vi "ISO8601 TimeString to Timestamp.vi"(9 "Strict ISO? (T)":bool=TRUE, 10 "Date (today)":timestamp, 11 "ISO8601 Time String":string) -> (1 "valid?":bool, 3 "Timestamp":timestamp)   [LabVIEW 2024]
uses:
  <vilib>/regexp/Match Regular Expression.xnode
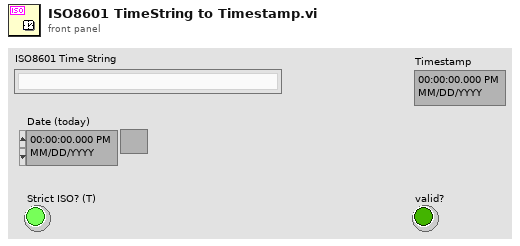
[diagram p1: front panel]
types:
  T1 = typedef "LVDateTimeRec.ctl" = cluster{"fractional second":dbl, "second":i32, "minute":i32, "hour":i32, "day of month":i32, "month":i32, "year":i32, "day of week":i32, "day of year":i32, "DST":i32}
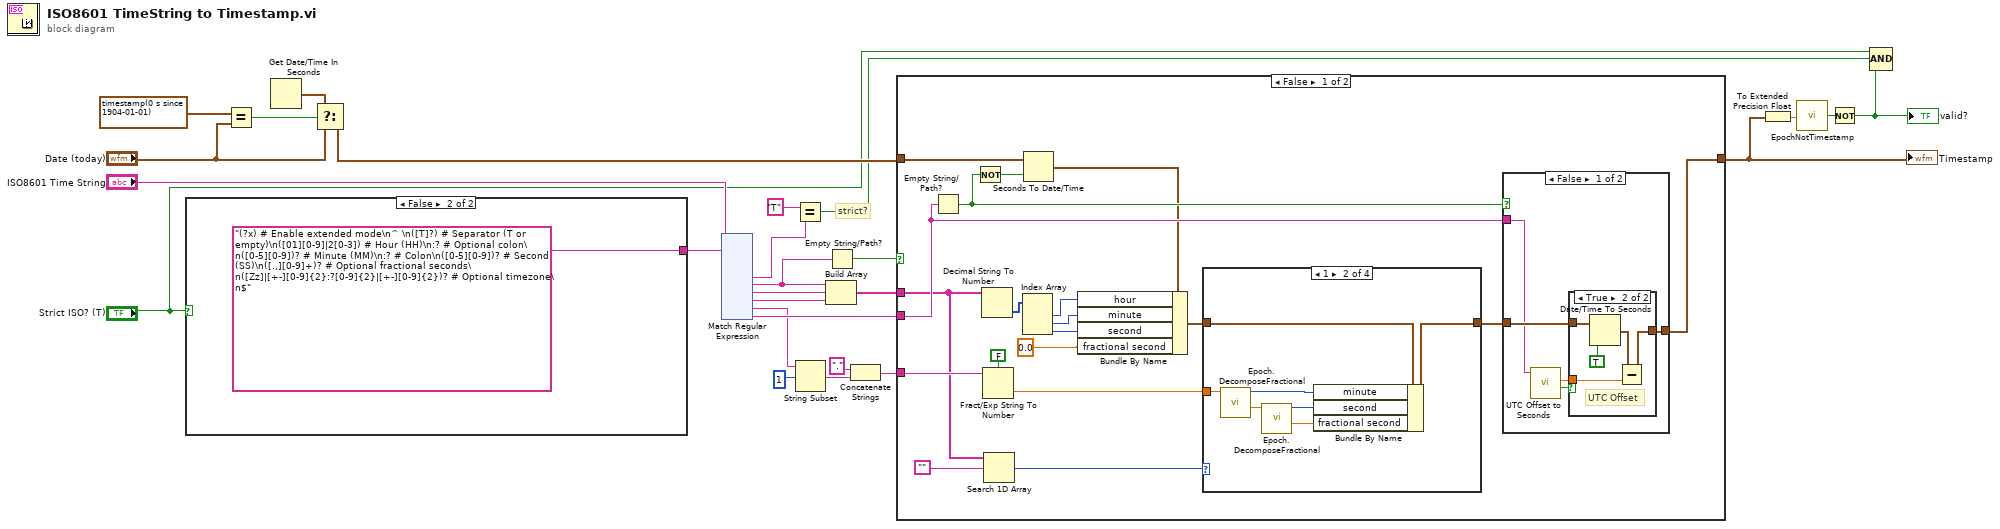
[diagram p0: block diagram]
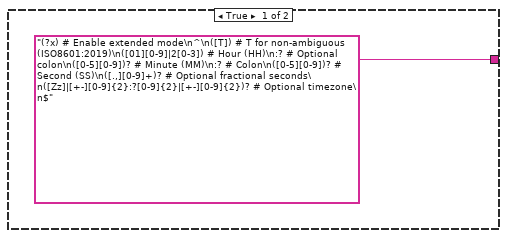
[diagram p2: hidden frame]
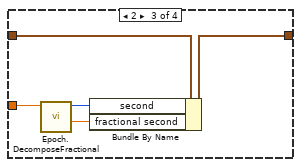
[diagram p4: hidden frame]
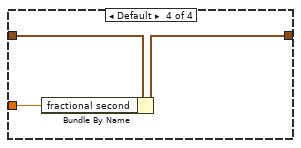
[diagram p5: hidden frame]
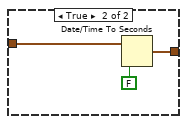
[diagram p7: hidden frame]
diagram:
  # "strict?"
  n1 = case shown="False" "Strict ISO? (T)" {
    tunnel: ["(?x) # Enable extended mode\n^\n([T]) # T for non-ambiguous (ISO8601:2019)\n([01][0-9]|2[0-3]) # Hour (HH)\n:? # Optional colon\n([0-5][0-9])? # Minute (MM)\n:? # Colon\n([0-5][0-9])? # Second (SS)\n([.,][0-9]+)? # Optional fractional seconds\n([Zz]|[+-][0-9]{2}:?[0-9]{2}|[+-][0-9]{2})? # Optional timezone\n$" ("regular expression") "(?x) # Enable extended mode\n^ \n([T]?) # Separator (T or empty)\n([01][0-9]|2[0-3]) # Hour (HH)\n:? # Optional colon\n([0-5][0-9])? # Minute (MM)\n:? # Colon\n([0-5][0-9])? # Second (SS)\n([.,][0-9]+)? # Optional fractional seconds\n([Zz]|[+-][0-9]{2}:?[0-9]{2}|[+-][0-9]{2})? # Optional timezone\n$" ("regular expression")] -> w7
    frame True {
    }
    frame False {
    }
  }
  n2 = Equal?(x=timestamp(0 s since 1904-01-01), y="Date (today)") -> (x = y?=w13:bool)
  n3 = Get Date/Time In Seconds() -> (seconds since 1Jan1904=w10:timestamp)
  n4 = Select(t=w10, s=w13, f="Date (today)") -> (s? t:f=w11:timestamp)
  n5 = xnode "Match Regular Expression"("input string"="ISO8601 Time String", "regular expression"=w7) -> ("submatch 1"=w9:string, "submatch 2"=w5:string, "submatch 3"=w22:string, "submatch 4"=w21:string, "submatch 5"=w16:string, "submatch 6"=w20:string)  [unwired: 4 in, 5 out]
  n6 = Equal?(x="T", y=w9) -> (x = y?=w3:bool)
  n7 = String Subset(string=w16, offset (0)=1 ("length (len. of substring)")) -> (substring=w17:string)  [unwired: 1 in]
  n8 = Build Array(w5, w22, w21) -> (w6:string[])
  n9 = Empty String/Path?(string/path=w5) -> (empty?=w4:bool)
  n10 = Concatenate Strings("." ("substring (\"\")"), w17) -> (w15:string)
  n11 = case shown="False" w4 {
    tunnel: w15 -> [w47 _]
    tunnel: w6 -> [w35 _]
    tunnel: w20 -> [w38 _]
    tunnel: w11 -> [w41 _]
    tunnel: [w29 _] -> w24
    frame False {
      n12 = Empty String/Path?(string/path=w38) -> (empty?=w42:bool)
      n13 = Not(x=w42) -> (.not. x?=w39:bool)
      n14 = Decimal String To Number(string=w35) -> (number=w40:i32[])  [unwired: 2 in, 1 out]
      n15 = Fract/Exp String To Number(use system decimal point (T)=FALSE, string=w47) -> (number=w30:dbl)  [unwired: 2 in, 1 out]
      n16 = Search 1D Array(1D array=w35, element="") -> (index of element=w33:i32)  [unwired: 1 in]
      n17 = Index Array(array=w40) -> (element #1=w44:i32, element #2=w45:i32, element #3=w46:i32)  [unwired: 3 in]
      n18 = Seconds To Date/Time(time stamp (now)=w41, to UTC (F)=w39) -> (date time rec=w37:T1)
      n19 = Bundle By Name(cluster=w37, "hour"=w44, "minute"=w45, "second"=w46, "fractional second"=0.0) -> (w32:T1)
      n20 = case shown="1" w33 {
        tunnel: w32 -> [w48 w55 w60 w63]
        tunnel: [w48 w54 w59 w62] -> w31
        tunnel: w30 -> [_ w53 w58 w61]
        frame 0 {
          # "This case cannot\neven be called. It would mean\nthat the HOUR is empty."
        }
        frame 1 {
          n21 = call "Epoch.DecomposeFractional.vi"("Fractional in"=w53) -> ("Fractional"=w50:dbl, "Integer"=w52:i32)  [unwired: 9 in]
          n22 = call "Epoch.DecomposeFractional.vi"("Fractional in"=w50) -> ("Fractional"=w49:dbl, "Integer"=w51:i32)  [unwired: 9 in]
          n23 = Bundle By Name(cluster=w55, "minute"=w52, "second"=w51, "fractional second"=w49) -> (w54:T1)
        }
        frame 2 {
          n24 = call "Epoch.DecomposeFractional.vi"("Fractional in"=w58) -> ("Fractional"=w56:dbl, "Integer"=w57:i32)  [unwired: 9 in]
          n25 = Bundle By Name(cluster=w60, "second"=w57, "fractional second"=w56) -> (w59:T1)
        }
        frame Default {
          n26 = Bundle By Name(cluster=w63, "fractional second"=w61) -> (w62:T1)
        }
      }
      n27 = case shown="False" w42 {
        tunnel: w31 -> [w66 w76]
        tunnel: [w65 w74] -> w29
        tunnel: w38 -> [w64 _]
        frame False {
          n28 = call "UTC Offset to Seconds.vi"("UTC Offset String"=w64) -> ("Valid?"=w68:bool, "Offset (s)"=w67:ext)  [unwired: 7 in, 2 out]
          n29 = case shown="True" w68 {
            tunnel: w66 -> [_ w72]
            tunnel: w67 -> [_ w71]
            tunnel: [_ w69] -> w65
            frame False {
            }
            frame True {
              # "UTC Offset"
              n30 = Date/Time To Seconds(1:TRUE ("is UTC (F)"), 2:w72) -> (0:w70:timestamp)
              n31 = Subtract(x=w70, y=w71) -> (x-y=w69:timestamp)
            }
          }
        }
        frame True {
          n32 = Date/Time To Seconds(1:FALSE ("is UTC (F)"), 2:w76) -> (0:w74:timestamp)
        }
      }
    }
    frame True {
    }
  }
  "Timestamp" <- w24
  n33 = To Extended Precision Float(1:w24) -> (0:w26:ext)
  n34 = call "EpochNotTimestamp.vi"("Epoch Time"=w26) -> ("Not a Timestamp?"=w25:bool)  [unwired: 8 in]
  n35 = Not(x=w25) -> (.not. x?=w1:bool)
  "valid?" <- w1
  n36 = Compound Arithmetic op=AND("Strict ISO? (T)", w3, w1) -> ()  [unwired: 1 out]
